vi "NF LI56xx u_crackToParamArray.vi"(0 "answerParam":string, 1 "delimiter":string=",") -> (14 "paramArray":string[](array[string]))   [LabVIEW 2019]
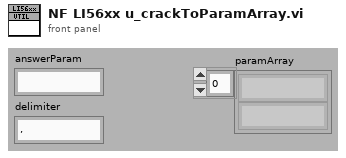
[diagram p1: front panel]
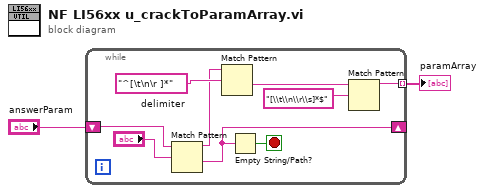
[diagram p0: block diagram]
diagram:
  n1 = while {
    tunnel: [w5] -> w1 mode=indexing
    shift-right: [w4] -> _
    shift-left: "answerParam" -> [w11]
    stop <- w3 stop-if-true
    n2 = Match Pattern(string=w11, regular expression="delimiter") -> (before substring=w8:string, after substring=w4:string)  [unwired: 1 in, 2 out]
    n3 = Match Pattern(string=w8, regular expression="^[\t\n\r ]*" ("正規表現")) -> (after substring=w7:string)  [unwired: 1 in, 3 out]
    n4 = Empty String/Path?(string/path=w4) -> (empty?=w3:bool)
    n5 = Match Pattern(string=w7, regular expression="[\\t\\n\\r\\s]*$" ("正規表現")) -> (before substring=w5:string)  [unwired: 1 in, 3 out]
  }
  "paramArray" <- w1
